vi "findCom.vi"(8 "error in (no error)":errorcluster, 11 "GiaoTiep in":refnum<class "GiaoTiepUART.lvclass">) -> (0 "error out":errorcluster, 3 "GiaoTiep out":refnum<class "GiaoTiepUART.lvclass">)   [LabVIEW 2017, in "LibraryGcode.lvlib" / "GiaoTiepUART.lvclass"]
uses:
  GiaoTiepUART.lvclass
  <vilib>/Instr/_visa.llb/VISA Find Search Mode.ctl
  GiaoTiepUART.lvclass/GiaoTiepUART.ctl
  <vilib>/Instr/_visa.llb/VISA Configure Serial Port (Instr).vi
panel:
  in  "termination char\n(0xA = '\\n' = LF)":u8=10 format="%.0x"
  out "StateError":bool
  out "OUT COM":refnum<visa-resource-name>
  out "CONNECT OK":bool
  out "find list":string[](array[string])
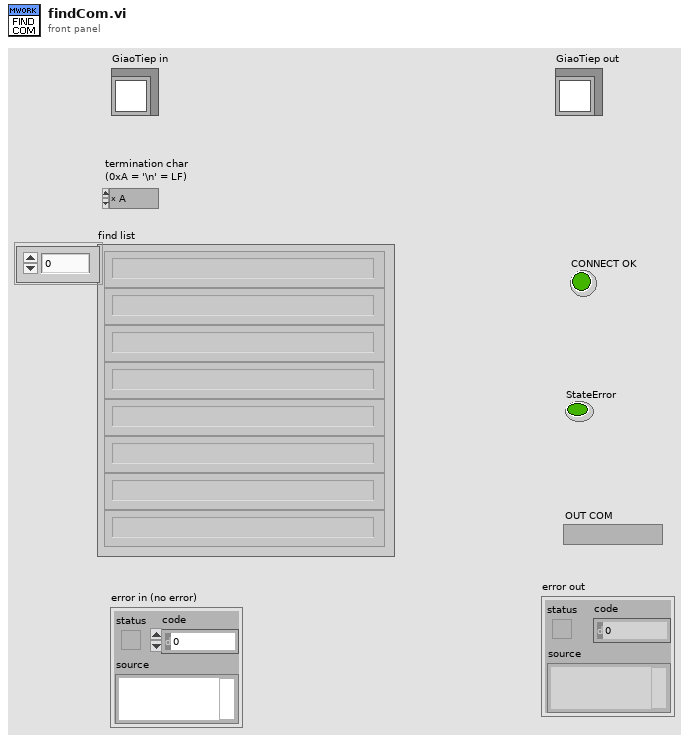
[diagram p1: front panel]
types:
  T1 = enum16{"InitCOM", "WriteCheck", "ReadCheck", "Comparedata", "End", "Stop"}
  T2 = typedef "VISA Find Search Mode.ctl" = u32
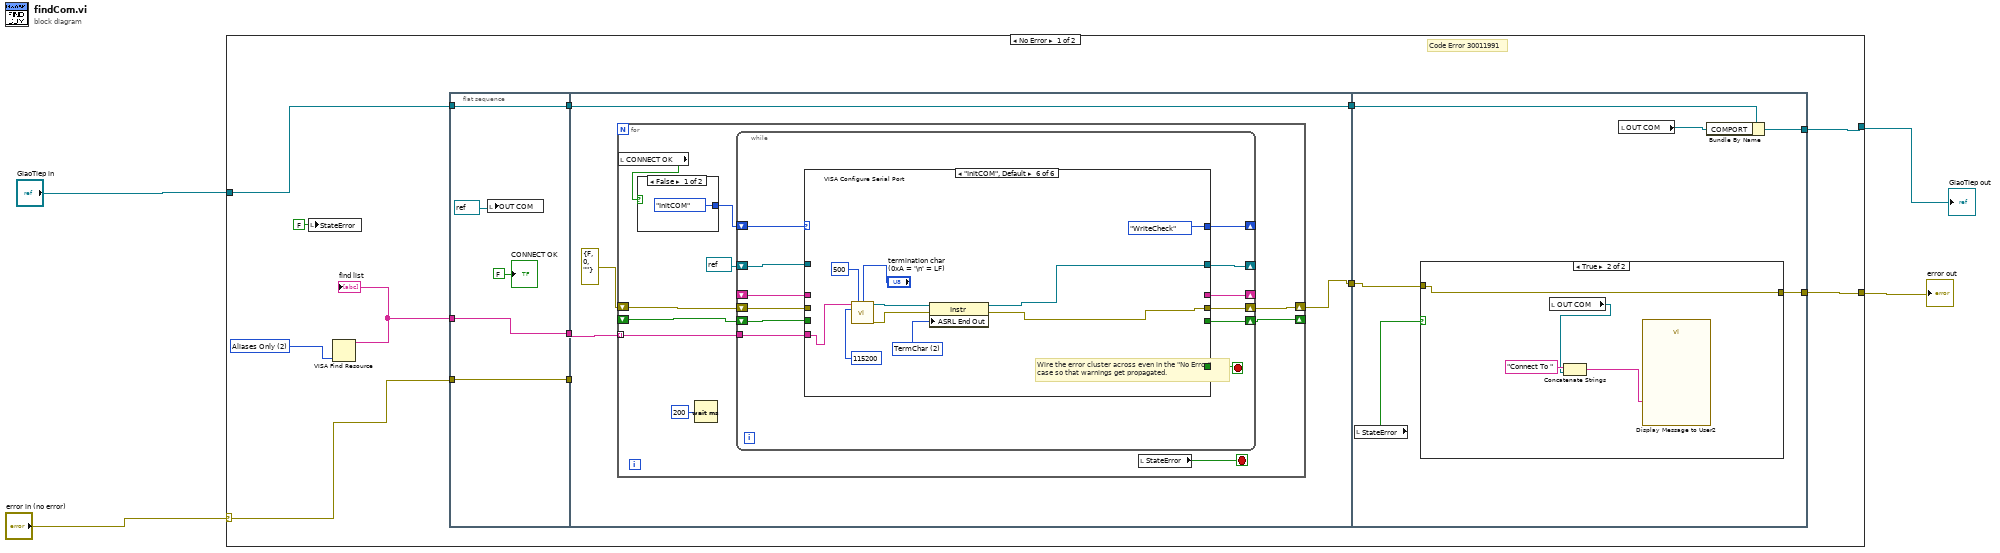
[diagram p0: block diagram]
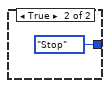
[diagram p2: hidden frame]
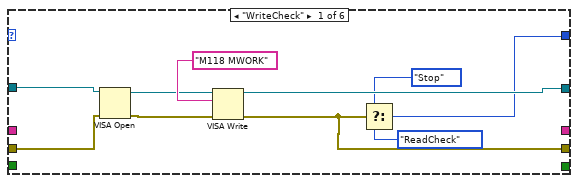
[diagram p3: hidden frame]
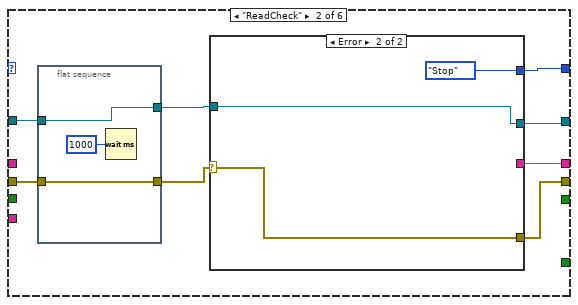
[diagram p4: hidden frame]
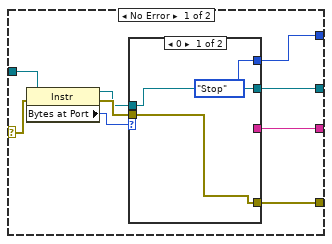
[diagram p5: hidden frame]
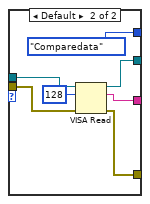
[diagram p6: hidden frame]
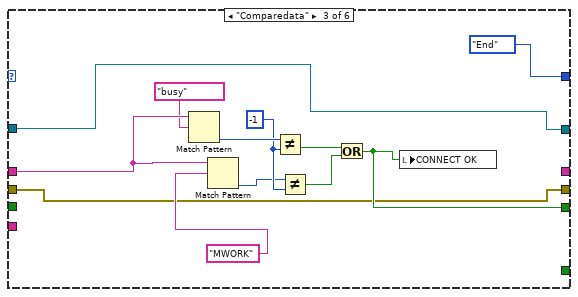
[diagram p7: hidden frame]
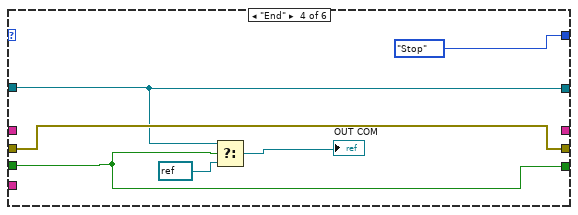
[diagram p8: hidden frame]
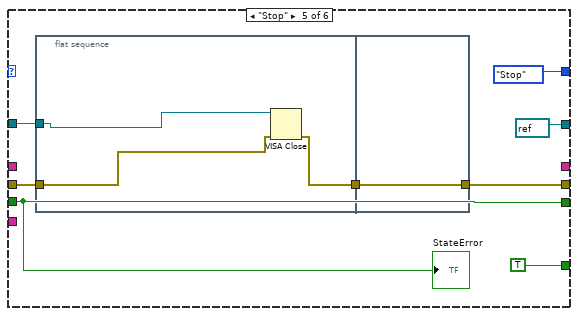
[diagram p9: hidden frame]
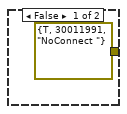
[diagram p10: hidden frame]
diagram:
  n1 = case shown="No Error" "error in (no error)" {
    selector: "error in (no error)" -> [w10 w145]
    tunnel: [w9 w145] -> w3
    tunnel: [w5 w144] -> w1
    tunnel: "GiaoTiep in" -> [w7 w144]
    frame No Error {
      w13 = T2 2 items=["Canonical Names Only"=0, "Aliases Only"=2, "Include Matching Aliases"=3, "Include All Aliases"=4] ("Search Mode")
      # "Code Error 30011991"
      # "Wire the error cluster across even in the \"No Error\"\ncase so that warnings get propagated."
      n2 = local write "StateError"(FALSE ("Boolean")) -> ()
      n3 = VISA Find Resource(10:w13) -> (3:w12:string[])  [unwired: 2 in, 2 out]
      "find list" <- w12
      n4 = flat-sequence {
        tunnel: w10 -> [w20]
        tunnel: w12 -> [w21]
        tunnel: [w21] -> w16
        tunnel: [w20] -> w15
        tunnel: [w17] -> w8
        tunnel: w7 -> [w17]
        tunnel: [w22] -> w14
        tunnel: w16 -> [w25]
        tunnel: w15 -> [_]
        tunnel: w8 -> [w23]
        tunnel: [w23] -> w6
        tunnel: w14 -> [w137]
        tunnel: [w136] -> w9
        tunnel: w6 -> [w135]
        tunnel: [w133] -> w5
        frame #0 {
          n5 = local write "OUT COM"(refnum<visa-resource-name> refnum ("f")) -> ()
          "CONNECT OK" <- FALSE ("CONNECT OK")
        }
        frame #1 {
          n6 = for {
            tunnel: w25 -> [w33] mode=indexing
            shift-right: [w28] -> _
            shift-left: _ -> [w29]
            shift-right: [w35] -> w22
            shift-left: errorcluster {"status"=FALSE, "code"=0, "source"=""} ("error out") -> [w32]
            stop <- w30 stop-if-true
            n7 = local read "CONNECT OK"() -> (w27:bool)
            n8 = case shown="False" w27 {
              tunnel: [T1."InitCOM" ("State") T1."Stop" ("State")] -> w26
              frame False {
              }
              frame True {
              }
            }
            n9 = Wait (ms)(milliseconds to wait=u32 200) -> ()  [unwired: 1 out]
            n10 = while {
              shift-right: [w39] -> _
              shift-left: w26 -> [w49]
              shift-right: [w41] -> _
              shift-left: refnum<visa-resource-name> refnum ("VISA resource name out") -> [w48]
              shift-right: [w46] -> w35
              shift-left: w32 -> [w47]
              shift-right: [w45] -> _
              shift-left: _ -> [w44]
              shift-right: [w43] -> w28
              shift-left: w29 -> [w42]
              tunnel: w33 -> [w38]
              stop <- w40 stop-if-true
              n11 = case shown="\"InitCOM\", Default" w49 {
                tunnel: w48 -> [w56 w62 w96 w105 w115 _]
                tunnel: [w59 w66 w96 w105 refnum<visa-resource-name> refnum ("VISA resource name out") w124] -> w41
                tunnel: w47 -> [w57 w61 w93 w109 w116 _]
                tunnel: [w50 w67 w93 w109 w117 w123] -> w46
                tunnel: [_ w65 _ _ _ _] -> w45
                tunnel: w44 -> [_ _ w102 _ _ _]
                tunnel: [_ _ w94 w108 w112 _] -> w43
                tunnel: w42 -> [_ _ _ w108 w112 _]
                tunnel: [_ _ _ _ TRUE _] -> w40
                tunnel: [w53 w64 T1."End" ("State") T1."Stop" ("State") T1."Stop" ("State") T1."WriteCheck" ("State")] -> w39
                tunnel: w38 -> [_ _ _ _ _ w125]
                frame "WriteCheck" {
                  n12 = VISA Open(error in (no error)=w57, VISA resource name=w56) -> (VISA resource name=w54:refnum<visa-resource-name>, error out=w55:errorcluster)  [unwired: 3 in]
                  n13 = VISA Write(VISA resource name=w54, write buffer="M118 MWORK" ("string"), error in (no error)=w55) -> (VISA resource name out=w59:refnum<visa-resource-name>, error out=w50:errorcluster)  [unwired: 1 out]
                  n14 = Select(t=T1."Stop" ("f"), s=w50, f=T1."ReadCheck" ("State")) -> (s? t:f=w53:T1)
                }
                frame "ReadCheck" {
                  n15 = flat-sequence {
                    tunnel: [w70] -> w63
                    tunnel: w62 -> [w70]
                    tunnel: [w69] -> w60
                    tunnel: w61 -> [w69]
                    frame #0 {
                      n16 = Wait (ms)(milliseconds to wait=u32 1000) -> ()  [unwired: 1 out]
                    }
                  }
                  n17 = case shown="Error" w60 {
                    selector: w60 -> [w71 w90]
                    tunnel: [w75 w90] -> w67
                    tunnel: w63 -> [w79 w91]
                    tunnel: [w76 w91] -> w66
                    tunnel: [w74 _] -> w65
                    tunnel: [w73 T1."Stop" ("State")] -> w64
                    frame No Error {
                      n18 = property class="Instr"(reference=w79, error in=w71) -> (reference out=w77:refnum<visa-resource-name>, error out=w78:errorcluster, "Bytes at Port"=w72:u32)
                      n19 = case shown="0" w72 {
                        tunnel: w78 -> [w80 w89]
                        tunnel: w77 -> [w81 w88]
                        tunnel: [w81 w87] -> w76
                        tunnel: [w80 w86] -> w75
                        tunnel: [_ w85] -> w74
                        tunnel: [T1."Stop" ("State") T1."Comparedata" ("State")] -> w73
                        frame 0 {
                        }
                        frame Default {
                          n20 = VISA Read(VISA resource name=w88, byte count=u32 128, error in (no error)=w89) -> (VISA resource name out=w87:refnum<visa-resource-name>, read buffer=w85:string, error out=w86:errorcluster)  [unwired: 1 out]
                        }
                      }
                    }
                    frame Error {
                    }
                  }
                }
                frame "Comparedata" {
                  w99 = -1 ("y")
                  n21 = Match Pattern(string=w102, regular expression="busy") -> (offset past match=w100:i32)  [unwired: 1 in, 3 out]
                  n22 = Match Pattern(string=w102, regular expression="MWORK" ("search string")) -> (offset past match=w95:i32)  [unwired: 1 in, 3 out]
                  n23 = Not Equal?(x=w100, y=w99) -> (x != y?=w98:bool)
                  n24 = Not Equal?(x=w95, y=w99) -> (x != y?=w97:bool)
                  n25 = Or(x=w98, y=w97) -> (x .or. y?=w94:bool)
                  n26 = local write "CONNECT OK"(w94) -> ()
                }
                frame "End" {
                  n27 = Select(t=w105, s=w108, f=refnum<visa-resource-name> refnum) -> (s? t:f=→"OUT COM":refnum<visa-resource-name>)
                }
                frame "Stop" {
                  n28 = flat-sequence {
                    tunnel: w116 -> [w119]
                    tunnel: w115 -> [w120]
                    tunnel: [w121] -> w113
                    tunnel: [w122] -> w117
                    tunnel: w113 -> [w122]
                    frame #0 {
                      n29 = VISA Close(VISA resource name=w120, error in (no error)=w119) -> (error out=w121:errorcluster)
                    }
                    frame #1 {
                    }
                  }
                  "StateError" <- w112
                }
                frame "InitCOM", Default {
                  w131 = u16 2 items=["None", "Last Bit", "TermChar", "Break"] ("Serial Settings:End Mode for Writes")
                  n30 = call-poly "VISA Configure Serial Port"("VISA resource name"=w125, "timeout (10sec)"=u32 500, "termination char\n(0xA = '\\n' = LF)"="termination char\n(0xA = '\\n' = LF)", "baud rate (9600)"=u32 115200) -> ("VISA resource name out"=w129:refnum<visa-resource-name>, "error out"=w130:errorcluster)  [unwired: 10 in]
                  n31 = property class="Instr"(reference=w129, error in=w130, "ASRL End Out"=w131) -> (reference out=w124:refnum<visa-resource-name>, error out=w123:errorcluster)
                }
              }
            }
            n32 = local read "StateError"() -> (w30:bool)
          }
        }
        frame #2 {
          n33 = local read "StateError"() -> (w138:bool)
          n34 = case shown="True" w138 {
            tunnel: w137 -> [_ w140]
            tunnel: [errorcluster {"status"=TRUE, "code"=30011991, "source"="NoConnect "} ("error out") w140] -> w136
            frame False {
            }
            frame True {
              n35 = local read "OUT COM"() -> (w141:refnum<visa-resource-name>)
              n36 = Concatenate Strings("Connect To " ("string"), w141) -> (w143:string)
              n37 = call "Display Message to User2"("Message"=w143) -> ()  [unwired: 9 in, 2 out]
            }
          }
          n38 = local read "OUT COM"() -> (w134:refnum<visa-resource-name>)
          n39 = Bundle By Name(cluster=w135, "COMPORT"=w134) -> (w133:refnum<class "GiaoTiepUART.lvclass">)
        }
      }
    }
    frame Error {
    }
  }
  "error out" <- w3
  "GiaoTiep out" <- w1
